vi "AddTestMethod_Provider_OnCommand.vi"(10 "Command ID":string, 11 "objects":T1[](array[typedef])) -> ()   [LabVIEW 2013]
uses:
  <resource>/Framework/Providers/API/ItemRef.ctl
panel:
  out "error out":errorcluster
  in  "error in":errorcluster
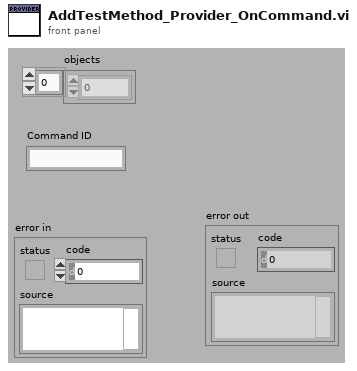
[diagram p1: front panel]
types:
  T1 = typedef "ItemRef.ctl" = u64
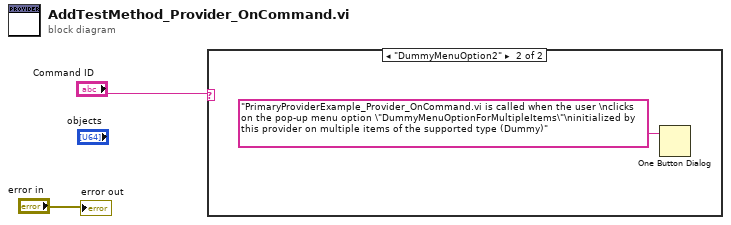
[diagram p0: block diagram]
diagram:
  n1 = case shown="\"DummyMenuOption2\"" "Command ID" {
    frame Default {
    }
    frame "DummyMenuOption2" {
      n2 = One Button Dialog(message="PrimaryProviderExample_Provider_OnCommand.vi is called when the user \nclicks on the pop-up menu option \"DummyMenuOptionForMultipleItems\"\ninitialized by this provider on multiple items of the supported type (Dummy)") -> ()  [unwired: 1 in, 1 out]
    }
  }
  "error out" <- "error in"
